vi "Digilens DLP Gen2 UI .vi"(11 "TopLevel In":refnum<class "TopLevel.lvclass">) -> (3 "TopLevel Out":refnum<class "TopLevel.lvclass">)   [LabVIEW 2022 SP3, in "TopLevel.lvclass"] (continued)
            n1054 = Unbundle By Name(w3179) -> ("Materials"=w3165:string[], "Color Panes"=w3163:string[], "DLP2Config.ColorPaneMapping.Head 1.Material"=w3178:string, "DLP2Config.ColorPaneMapping.Head 1.ColorPane"=w3172:string, "DLP2Config.ColorPaneMapping.Head 2.Material"=w3177:string, "DLP2Config.ColorPaneMapping.Head 2.ColorPane"=w3171:string, "DLP2Config.ColorPaneMapping.Head 3.Material"=w3176:string, "DLP2Config.ColorPaneMapping.Head 3.ColorPane"=w3170:string, "DLP2Config.ColorPaneMapping.Head 4.Material"=w3175:string, "DLP2Config.ColorPaneMapping.Head 4.ColorPane"=w3169:string, "DLP2Config.ColorPaneMapping.Head 5.Material"=w3174:string, "DLP2Config.ColorPaneMapping.Head 5.ColorPane"=w3168:string, "DLP2Config.ColorPaneMapping.Head 6.Material"=w3173:string, "DLP2Config.ColorPaneMapping.Head 6.ColorPane"=w3167:string)
            n1055 = Build Array(w3172, w3171, w3170, w3169, w3168, w3167) -> (w3164:string[])
            n1056 = Build Array(w3178, w3177, w3176, w3175, w3174, w3173) -> (w3166:string[])
            n1057 = for {
              tunnel: w3166 -> [w3189] mode=indexing
              tunnel: w3165 -> [w3188]
              tunnel: [w3186] -> w3161 mode=indexing
              n1058 = Search 1D Array(1D array=w3188, element=w3189) -> (index of element=w3187:i32)  [unwired: 1 in]
              n1059 = Greater Than 0?(x=w3187) -> (x > 0?=w3186:bool)
            }
            n1060 = for {
              tunnel: w3164 -> [w3185] mode=indexing
              tunnel: w3163 -> [w3184]
              tunnel: [w3182] -> w3162 mode=indexing
              n1061 = Search 1D Array(1D array=w3184, element=w3185) -> (index of element=w3183:i32)  [unwired: 1 in]
              n1062 = Greater Than 0?(x=w3183) -> (x > 0?=w3182:bool)
            }
            n1063 = And Array Elements(Boolean array=w3161) -> (logical AND=w3159:bool)
            n1064 = And Array Elements(Boolean array=w3162) -> (logical AND=w3160:bool)
            n1065 = case shown="True" w3160 {
              frame False {
              }
              frame True {
                n1066 = One Button Dialog(message="Atleast 1 material  mismatch\nbetween DB and Config") -> ()  [unwired: 1 in, 1 out]
              }
            }
            n1067 = case shown="True" w3159 {
              frame False {
              }
              frame True {
                n1068 = One Button Dialog(message="Atleast 1 ColorPlane  mismatch\nbetween DB and Config") -> ()  [unwired: 1 in, 1 out]
              }
            }
          }
          frame Enabled {
          }
        }
        n1069 = call <vilib>:"Add State(s) to Queue__JKI_lib_State_Machine.vi"("State(s) in (\"\")"=w3158) -> ("States Out"=w3157:string)  [unwired: 14 in]
      }
      frame "Data: GetMaterialsAndColorPlanes" {
        w3195 = T18[] [enum."1", enum."2", enum."3", enum."4", enum."5", enum."6"] items=["-1", "1", "2", "3", "4", "5", "6"]
        n1070 = Unbundle By Name(w3202) -> ("DLP2Config.ColorPlanes"=w3196:string[], "DLP2Config.Materials"=w3197:string[], "Database"=w3201:refnum<class "Database.lvclass">, "TopLevel out"=w3194:refnum<class "TopLevel.lvclass">)
        n1071 = property class="TopLevel.lvclass" props=["Methods:Accessors:ConfigDict", "Methods:Accessors:PrinterInitializationXML"](reference=w3194) -> ("Methods:Accessors:PrinterInitializationXML"=w3193:T61)  [unwired: 1 in, 3 out]
        n1072 = Unbundle By Name(w3193) -> ("InkSet.Ink"=w3192:T65[])  [unwired: 1 out]
        n1073 = disable-structure shown="Enabled" {
          disable-tunnel: w3201 -> [w3219 _ _]
          disable-tunnel: [w3216 w3220 w3236] -> w3200
          disable-tunnel: w3199 -> [w3215 w3220 w3230]
          disable-tunnel: [w3208 w3221 w3235] -> w3190
          disable-tunnel: [w3207 w3222 _] -> _
          disable-tunnel: w3197 -> [_ w3222 _]
          disable-tunnel: w3196 -> [_ w3221 _]
          disable-tunnel: w3194 -> [_ _ w3233]
          disable-tunnel: w3195 -> [_ _ w3237]
          disable-tunnel: w3192 -> [_ _ w3234]
          disable-tunnel: [_ _ w3231] -> w3191
          frame Disabled {
            w3213 = u32 3000 ("Timeout (ms)")
            w3214 = TRUE ("Wait (F)")
            n1074 = call "API_DB.GetAllMaterials.vi"("Database in"=w3219, "Wait (F)"=w3214, "error in (no error)"=w3215, "Timeout (ms)"=w3213) -> ("Database out"=w3218:refnum<class "Database.lvclass">, "Materials"=w3212:string[], "error out"=w3217:errorcluster)  [unwired: 9 in]
            n1075 = call "API_DB.GetAllColors.vi"("Database in"=w3218, "Wait (F)"=w3214, "error in (no error)"=w3217, "Timeout (ms)"=w3213) -> ("ColorPlanes"=w3209:string[], "error out"=w3216:errorcluster)  [unwired: 9 in, 1 out]
            n1076 = Build Array (concatenate)("none", w3212) -> (w3207:string[])
            n1077 = Build Array (concatenate)("none", w3209) -> (w3208:string[])
          }
          frame Disabled {
          }
          frame Enabled {
            n1078 = for {
              shift-right: [w3244] -> w3232
              shift-left: w3233 -> [w3245]
              shift-right: [w3242] -> w3236
              shift-left: w3230 -> [w3243]
              tunnel: [w3240] -> w3235 mode=indexing
              tunnel: w3234 -> [w3239] mode=indexing
              tunnel: [w3238] -> w3231 mode=indexing
              n1079 = Unbundle By Name(w3239) -> ("#attributes.InkType"=w3238:string)
              n1080 = call "GetMaterialPropertiesInConfigDict.vi"("error in (no error)"=w3243, "MaterialName"=w3238, "TopLevel in"=w3245) -> ("error out"=w3242:errorcluster, "Cluster"=w3241:T85, "TopLevel out"=w3244:refnum<class "TopLevel.lvclass">)  [unwired: 6 in]
              n1081 = Unbundle By Name(w3241) -> ("Ink.#attributes.ColorPlane"=w3240:string)
            }
            n1082 = property on="Head 4 Material" class="Ring (strict)"("Strings []"=w3231) -> ()  [unwired: 2 in, 2 out]
            n1083 = property on="Head 1 Material" class="Ring (strict)"("Strings []"=w3231) -> ()  [unwired: 2 in, 2 out]
            n1084 = property on="Head 5 Material" class="Ring (strict)"("Strings []"=w3231) -> ()  [unwired: 2 in, 2 out]
            n1085 = property on="Head 2 Material" class="Ring (strict)"("Strings []"=w3231) -> ()  [unwired: 2 in, 2 out]
            n1086 = property on="Head 6 Material" class="Ring (strict)"("Strings []"=w3231) -> ()  [unwired: 2 in, 2 out]
            n1087 = property on="Head 3 Material" class="Ring (strict)"("Strings []"=w3231) -> ()  [unwired: 2 in, 2 out]
            n1088 = property on="Head 4 Material 2" class="Ring (strict)"("Strings []"=w3231) -> ()  [unwired: 2 in, 2 out]
            n1089 = property on="Head 6 Material 2" class="Ring (strict)"("Strings []"=w3231) -> ()  [unwired: 2 in, 2 out]
            n1090 = property on="Head 1 Material 2" class="Ring (strict)"("Strings []"=w3231) -> ()  [unwired: 2 in, 2 out]
            n1091 = property on="Head 2 Material 2" class="Ring (strict)"("Strings []"=w3231) -> ()  [unwired: 2 in, 2 out]
            n1092 = property on="Head 3 Material 2" class="Ring (strict)"("Strings []"=w3231) -> ()  [unwired: 2 in, 2 out]
            n1093 = property on="Head 5 Material 2" class="Ring (strict)"("Strings []"=w3231) -> ()  [unwired: 2 in, 2 out]
            n1094 = for {
              shift-right: [w3254] -> _
              shift-left: w3232 -> [w3255]
              tunnel: w3237 -> [w3250] mode=indexing
              shift-right: [w3252] -> _
              shift-left: _ -> [w3253]
              tunnel: w3231 -> [w3249]
              tunnel: [w3247] -> _ mode=indexing
              tunnel: [w3246] -> w3229 mode=indexing
              n1095 = call "GetHeadPropertiesInConfigDict.vi"("error in (no error)"=w3253, "#attributes.HeadNumber"=w3250, "TopLevel in"=w3255) -> ("error out"=w3252:errorcluster, "HeadProperties"=w3251:T63, "TopLevel out"=w3254:refnum<class "TopLevel.lvclass">)  [unwired: 6 in]
              n1096 = Unbundle By Name(w3251) -> ("#attributes.Material"=w3248:string)
              n1097 = Search 1D Array(1D array=w3249, element=w3248) -> (index of element=w3246:i32)  [unwired: 1 in]
              n1098 = Greater Or Equal To 0?(x=w3246) -> (x >= 0?=w3247:bool)
            }
            n1099 = Index Array(array=w3229) -> (element #1=w3228:i32, element #2=w3227:i32, element #3=w3226:i32, element #4=w3225:i32, element #5=w3224:i32, element #6=w3223:i32)  [unwired: 6 in]
            n1100 = property on="Head 4 Material 2" class="Ring (strict)"("Value"=w3225) -> ()  [unwired: 2 in, 2 out]
            n1101 = property on="Head 6 Material 2" class="Ring (strict)"("Value"=w3223) -> ()  [unwired: 2 in, 2 out]
            n1102 = property on="Head 1 Material 2" class="Ring (strict)"("Value"=w3228) -> ()  [unwired: 2 in, 2 out]
            n1103 = property on="Head 2 Material 2" class="Ring (strict)"("Value"=w3227) -> ()  [unwired: 2 in, 2 out]
            n1104 = property on="Head 3 Material 2" class="Ring (strict)"("Value"=w3226) -> ()  [unwired: 2 in, 2 out]
            n1105 = property on="Head 5 Material 2" class="Ring (strict)"("Value"=w3224) -> ()  [unwired: 2 in, 2 out]
            n1106 = property on="Head 1 Material" class="Ring (strict)"("Value"=w3228) -> ()  [unwired: 2 in, 2 out]
            n1107 = property on="Head 2 Material" class="Ring (strict)"("Value"=w3227) -> ()  [unwired: 2 in, 2 out]
            n1108 = property on="Head 3 Material" class="Ring (strict)"("Value"=w3226) -> ()  [unwired: 2 in, 2 out]
            n1109 = property on="Head 4 Material" class="Ring (strict)"("Value"=w3225) -> ()  [unwired: 2 in, 2 out]
            n1110 = property on="Head 5 Material" class="Ring (strict)"("Value"=w3224) -> ()  [unwired: 2 in, 2 out]
            n1111 = property on="Head 6 Material" class="Ring (strict)"("Value"=w3223) -> ()  [unwired: 2 in, 2 out]
          }
        }
        n1112 = Bundle By Name(cluster=w3202, "DLP2Config.Materials"=w3191, "Color Panes"=w3190) -> (w3198:T77)
        n1113 = property on="Head 4 ColorPlane" class="Ring (strict)"("Strings []"=w3190) -> ()  [unwired: 2 in, 2 out]
        n1114 = property on="Head 1 ColorPlane" class="Ring (strict)"("Strings []"=w3190) -> ()  [unwired: 2 in, 2 out]
        n1115 = property on="Head 2 ColorPlane" class="Ring (strict)"("Strings []"=w3190) -> ()  [unwired: 2 in, 2 out]
        n1116 = property on="Head 3 ColorPlane" class="Ring (strict)"("Strings []"=w3190) -> ()  [unwired: 2 in, 2 out]
        n1117 = property on="Head 6 ColorPlane" class="Ring (strict)"("Strings []"=w3190) -> ()  [unwired: 2 in, 2 out]
        n1118 = property on="Head 5 ColorPlane" class="Ring (strict)"("Strings []"=w3190) -> ()  [unwired: 2 in, 2 out]
        n1119 = call <vilib>:"Add State(s) to Queue__JKI_lib_State_Machine.vi"("State(s) in (\"\")"=w3206) -> ("States Out"=w3205:string)  [unwired: 14 in]
      }
      frame "Data: Initialize" {
        w3256 = path[] []  # PPP_Ditherered_Images
        w3257 = FALSE  # PrePrimeTmrEnabled
        w3258 = TRUE  # PrePrimeDone
        w3260 = T75 {"UserLevel"=enum."Operator", "Login Time"=timestamp(0 s since 1904-01-01)}  # Login
        w3261 = T74 {"CellPrintRecipe"={"#attributes"={"Type"="", "RecipeName"="", "Product"=""}, "CellPrint"=[], "InkCompensationSet"={"InkCompensation"=[]}}}  # CalibrationPrints
        w3262 = T73 {"CellPrintRecipe"={"#attributes"={"Type"="", "RecipeName"="", "Product"=""}, "CellPrint"=[], "InkCompensationSet"={"InkCompensation"=[]}}}  # CurrentDLPRecipe
        w3263 = T71 {"PH1_Enable"=FALSE, "PH2_Enable"=FALSE, "PH3_Enable"=FALSE, "PH4_Enable"=FALSE, "PH5_Enable"=FALSE, "PH6_Enable"=FALSE}  # HeadStatusPollData
        w3269 = T49 {"Path_to_Tiff"=path "", "OutputFolder"=path "", "DPI_x"=0, "DPI_y"=0, "Python_Version"=enum."3.9 32"}  # SeparateLayers
        w3270 = T68 {"Path"=path "", "Type"="", "Product"=""}  # PrintDesign
        w3271 = cluster{"RecipeXMLPath":path} {"RecipeXMLPath"=path ""}  # Print
        w3275 = T71 {"PH1_Enable"=FALSE, "PH2_Enable"=FALSE, "PH3_Enable"=FALSE, "PH4_Enable"=FALSE, "PH5_Enable"=FALSE, "PH6_Enable"=FALSE}  # HeadStatus
        w3276 = variant  # SettingsUpdate
        w3277 = T70[] []  # GISHeadStatus
        w3278 = T86 {"Head 1"={"Actual"=0.0, "Target"=0.0}, "Head 2"={"Actual"=0.0, "Target"=0.0}, "Head 3"={"Actual"=0.0, "Target"=0.0}, "Head 4"={"Actual"=0.0, "Target"=0.0}, "Head 5"={"Actual"=0.0, "Target"=0.0}, "Head 6"={"Actual"=0.0, "Target"=0.0}}  # Head Temp
        w3279 = cluster{"HeaterEnblHead":T18, "Enable":bool} {"HeaterEnblHead"=enum."1", "Enable"=FALSE}  # Heater Enable
        w3282 = T69 {"ImageBufferMain"=[], "ChannelTargetMaterials"=[], "MaterialNames"=[]}  # TIFFImageData
        w3283 = T6 refnum  # Planes Image
        w3284 = T6 refnum  # RGB Image
        w3285 = refnum<class "DAQ.lvclass"> refnum  # DAQ
        w3294 = FALSE  # ConfigSaveRequired
        w3295 = string[] []  # Color Panes
        w3296 = string[] []  # Materials
        w3300 = refnum<class "DLP2.lvclass"> refnum  # DLP2
        w3299 = refnum<class "Database.lvclass"> refnum  # Database
        w3303 = API_Command_Enum."Execute Printer Commands"  # API Command
        w3304 = T67 {"GIS File Path"=path "", "Duration (s)"=0.1, "No. of Repeats"=1}  # Pre Purge Parameters
        w3305 = ICP1-D0_Channel_Names."None"  # Purge\PrePurge Channel Name
        w3312 = refnum<class "Motor Controller.lvclass"> refnum  # Motor Controller
        w3315 = refnum<class "GIS Printer.lvclass"> refnum  # GIS Printer
        w3317 = refnum<class "IO.lvclass"> refnum  # IO
        w3322 = T87 {"Current VI Reference"=refnum, "Close Panel on Exit?"=FALSE}  # Core
        n1120 = property class="TopLevel.lvclass"(reference=w3321) -> (reference out=w3309:refnum<class "TopLevel.lvclass">, "Methods:Accessors:IO"=w3319:refnum<class "IO.lvclass">, "Methods:Accessors:GIS Printer"=w3320:refnum<class "GIS Printer.lvclass">, "Methods:Accessors:Motor Controller"=w3314:refnum<class "Motor Controller.lvclass">, "Methods:Accessors:Digilens Config"=w3293:T51, "Methods:Accessors:PrinterInitializationXML"=w3274:T61, "Methods:Accessors:Database"=w3302:refnum<class "Database.lvclass">, "Methods:Accessors:DLP2"=w3301:refnum<class "DLP2.lvclass">, "Methods:Accessors:DLP2Config"=w3289:T35, "Methods:Accessors:DAQ"=w3287:refnum<class "DAQ.lvclass">, "Methods:Accessors:ConfigDict"=w3273:T16)  [unwired: 1 in, 1 out]
        n1121 = call-dynamic "GetEvents_TopLevel.vi"("error in (no error)"=w3307, "TopLevel in"=w3309) -> ("error out"=w3266:errorcluster, "UserEvents"=w3308:T88, "TopLevel out"=w3268:refnum<class "TopLevel.lvclass">)  [unwired: 7 in]
        n1122 = call-dynamic "Read PersistentXML.vi"("error in (no error)"=w3266, "TopLevel in"=w3268) -> ("error out"=w3265:errorcluster, "PersistentData"=w3264:T72, "TopLevel out"=w3267:refnum<class "TopLevel.lvclass">)  [unwired: 7 in]
        n1123 = Coerce To Type(0:w3289, 1:T35 {"Paths"={"DigiBit WG Design Folder"=path "", "Compensated GS Image Folder"=path "", "Nozzle GS Files Head 1"=path "", "Nozzle GS Files Head 2"=path "", "Nozzle GS Files Head 3"=path "", "Nozzle GS Files Head 4"=path "", "Nozzle GS Files Head 5"=path "", "Nozzle GS Files Head 6"=path ""}, "ColorPaneMapping"={"Head 1"={"Material"="", "ColorPane"=""}, "Head 2"={"Material"="", "ColorPane"=""}, "Head 3"={"Material"="", "ColorPane"=""}, "Head 4"={"Material"="", "ColorPane"=""}, "Head 5"={"Material"="", "ColorPane"=""}, "Head 6"={"Material"="", "ColorPane"=""}}, "Materials"=[], "ColorPlanes"=[], "SpitVoltages_Half"={"1"=0.0, "2"=0.0, "3"=0.0, "4"=0.0, "5"=0.0, "6"=0.0}, "SpitVoltages_Full"={"1"=0.0, "2"=0.0, "3"=0.0, "4"=0.0, "5"=0.0, "6"=0.0}, "SystemMode"=[], "PrimeModeConfig"=[], "Running Average Duration_s"=5.0} ("DLP2ConfigLoaded")) -> (2:w3288:T35)
        n1124 = Coerce To Type(0:w3289, 1:T35 {"Paths"={"DigiBit WG Design Folder"=path "", "Compensated GS Image Folder"=path "", "Nozzle GS Files Head 1"=path "", "Nozzle GS Files Head 2"=path "", "Nozzle GS Files Head 3"=path "", "Nozzle GS Files Head 4"=path "", "Nozzle GS Files Head 5"=path "", "Nozzle GS Files Head 6"=path ""}, "ColorPaneMapping"={"Head 1"={"Material"="", "ColorPane"=""}, "Head 2"={"Material"="", "ColorPane"=""}, "Head 3"={"Material"="", "ColorPane"=""}, "Head 4"={"Material"="", "ColorPane"=""}, "Head 5"={"Material"="", "ColorPane"=""}, "Head 6"={"Material"="", "ColorPane"=""}}, "Materials"=[], "ColorPlanes"=[], "SpitVoltages_Half"={"1"=0.0, "2"=0.0, "3"=0.0, "4"=0.0, "5"=0.0, "6"=0.0}, "SpitVoltages_Full"={"1"=0.0, "2"=0.0, "3"=0.0, "4"=0.0, "5"=0.0, "6"=0.0}, "SystemMode"=[], "PrimeModeConfig"=[], "Running Average Duration_s"=5.0} ("DLP2Config")) -> (2:w3291:T35)
        n1125 = Unbundle By Name(w3308) -> ("Exit Event"=w3306:refnum<user-event>)
        n1126 = Coerce To Type(0:w3319, 1:w3317) -> (2:w3318:refnum<class "IO.lvclass">)
        n1127 = Coerce To Type(0:w3287, 1:w3285) -> (2:w3286:refnum<class "DAQ.lvclass">)
        n1128 = Coerce To Type(0:w3320, 1:w3315) -> (2:w3316:refnum<class "GIS Printer.lvclass">)
        n1129 = Coerce To Type(0:w3302, 1:w3299) -> (2:w3298:refnum<class "Database.lvclass">)
        n1130 = Coerce To Type(0:w3301, 1:w3300) -> (2:w3297:refnum<class "DLP2.lvclass">)
        n1131 = call "GetPrimeConfigKeys.vi"() -> ("Prime Names"=w3272:T89)  [unwired: 11 in]
        n1132 = Coerce To Type(0:w3314, 1:w3312) -> (2:w3313:refnum<class "Motor Controller.lvclass">)
        n1133 = call <vilib>:"Add State(s) to Queue__JKI_lib_State_Machine.vi"("State(s) in (\"\")"=w3325) -> ("States Out"=w3324:string)  [unwired: 14 in]
        n1134 = Bundle("Core"=w3322, "IO"=w3318, "GIS Printer"=w3316, "Motor Controller"=w3313, "Methods:Accessors:Digilens Config"=w3293, "Methods:Accessors:PrinterInitializationXML"=w3274, "Status"=T40 {"Motor Controller Config Data"={"Motor IP Addresss"="", "Current Position"=0, "Pulse_Per_mm"=0, "PrePrint"=[], "Load Position_mm"=0, "Laminate Position_mm"=0}, "Motor Controller Data"={"Enabled?"=FALSE}, "Stage Move"={"Current Step"="", "Move Data"=[]}, "Stage Busy?"=FALSE}, "Exit Event"=w3306, "Purge\\PrePurge Channel Name"=w3305, "Pre Purge Parameters"=w3304, "API Command"=w3303, "TopLevel out"=w3267, "Database"=w3298, "DLP2"=w3297, "DLP2Config"=w3291, "Materials"=w3296, "Color Panes"=w3295, "ConfigSaveRequired"=w3294, "DLP2ConfigLoaded"=w3288, "PrintDesign"=w3270, "DAQ"=w3286, "RGB Image"=w3284, "Planes Image"=w3283, "TIFFImageData"=w3282, "Image Resolution"=T34 {"X Resolution"=0, "Y Resolution"=0}, "Pre Purge API Data"=T27 {"Interval (s)"=0.1, "PurgeDuration (s)"=0.1, "Repeats"=0, "PrimingMode"=enum."Pre-Purge", "Head"=enum."1", "Frequency (Hz)"=0, "PrintWeight"=0.1}, "Prime Names"=w3272, "Heater Enable"=w3279, "Head Temp"=w3278, "GISHeadStatus"=w3277, "SettingsUpdate"=w3276, "HeadStatus"=w3275, "Methods:Accessors:ConfigDict"=w3273, "Print"=w3271, "SeparateLayers"=w3269, "PersistentData"=w3264, "HeadStatusPollData"=w3263, "CurrentDLPRecipe"=w3262, "CalibrationPrints"=w3261, "Login"=w3260, "PrintWeights"=T33 {"Weights 1"=0.3, "Weights 2"=0.3, "Weights 3"=0.3, "Weights 4"=0.3, "Weights 5"=0.3, "Weights 6"=0.3}, "PrePrimeDone"=w3258, "PrePrimeTmrEnabled"=w3257, "PPP_Ditherered_Images"=w3256) -> (w3323:T77)  [unwired: 1 in]
      }
      frame "Data: Create Images" {
        w3328 = T90 0 items=["Grayscale (U8)", "Grayscale (I16)", "Grayscale (SGL)", "Complex (CSG)", "RGB (U32)", "HSL (U32)", "RGB (U64)", "Grayscale (U16)"] ("Image Type")
        w3334 = T90 4 items=["Grayscale (U8)", "Grayscale (I16)", "Grayscale (SGL)", "Complex (CSG)", "RGB (U32)", "HSL (U32)", "RGB (U64)", "Grayscale (U16)"] ("Image Type")
        n1135 = call "IMAQ Create"("Image Name"="RGB_TIFF_Image", "Image Type"=w3334, "error in (no error)"=w3333) -> ("New Image"=w3331:T6, "error out"=w3330:errorcluster)  [unwired: 2 in]
        n1136 = call "IMAQ Create"("Image Name"="TIFF_Planes_Image" ("String"), "Image Type"=w3328, "error in (no error)"=w3330) -> ("New Image"=w3327:T6, "error out"=w3329:errorcluster)  [unwired: 2 in]
        n1137 = Bundle By Name(cluster=w3338, "RGB Image"=w3331, "Planes Image"=w3327) -> (w3332:T77)
      }
      frame "Data: Cleanup" {
        # "Cleanup any data and references, here.\n(this is called automatically, by the Macro: Exit)"
        n1138 = Unbundle By Name(w3346) -> ("Core.Current VI Reference"=w3349:refnum<vi>, "Planes Image"=w3343:T6, "RGB Image"=w3342:T6)
        n1139 = call "IMAQ Dispose"("Image"=w3342) -> ("error out"=w3340:errorcluster)  [unwired: 5 in]
        n1140 = call "IMAQ Dispose"("Image"=w3343) -> ("error out"=w3341:errorcluster)  [unwired: 5 in]
        n1141 = flat-sequence {
          tunnel: w3341 -> [_]
          tunnel: w3340 -> [_]
          frame #0 {
          }
        }
        n1142 = Close Reference(reference=w3349, error in (no error)=w3348) -> (error out=w3347:errorcluster)
        n1143 = call <vilib>:"Add State(s) to Queue__JKI_lib_State_Machine.vi"("State(s) in (\"\")"=w3351) -> ("States Out"=w3350:string)  [unwired: 14 in]
      }
      frame "---------- UI ----------" {
        n1144 = call <vilib>:"Add State(s) to Queue__JKI_lib_State_Machine.vi"("State(s) in (\"\")"=w3357) -> ("States Out"=w3356:string)  [unwired: 14 in]
      }
      frame "UI: Update Status" {
        n1145 = control-ref of="PrintStatus"() -> (w3359:refnum<vi>)
        n1146 = property class="Str"(reference=w3359, "Value"=w3358) -> ()  [unwired: 1 in, 2 out]
        n1147 = call <vilib>:"Add State(s) to Queue__JKI_lib_State_Machine.vi"("State(s) in (\"\")"=w3365) -> ("States Out"=w3364:string)  [unwired: 14 in]
      }
      frame "UI: PrimeHeadTimerInit" {
        n1148 = property on="EnableHeadPrimeTimer" class="Bool (strict)"("Value"=TRUE ("Value (Signaling)")) -> ()  [unwired: 2 in, 2 out]
        n1149 = call <vilib>:"Add State(s) to Queue__JKI_lib_State_Machine.vi"("State(s) in Front (\"\")"="Action: PrePrimeTimer>>Init\nUI: EnableControls>>PrimeHeads>>True\nUI: EnableControls>>Print PPP Image>>False" ("State(s) in Front (\"\")"), "State(s) in (\"\")"=w3373) -> ("States Out"=w3372:string)  [unwired: 13 in]
      }
      frame "UI: Process Head Enabled Mode" {
        n1150 = Unbundle By Name(w3383) -> ("TopLevel out"=w3376:refnum<class "TopLevel.lvclass">)
        n1151 = call "FindEnable_DisableStatus.vi"("TopLevel in"=w3376) -> ("error out"=w3381:errorcluster, "Array"=w3382:T91)  [unwired: 8 in, 1 out]
        n1152 = Index Array(array=w3382) -> (element #1=w3377:T45, element #2=w3378:T45, element #3=w3379:T45, element #4=w3380:T45, element #5=w3375:T45, element #6=w3374:T45)  [unwired: 6 in]
        n1153 = property on="PrinterControls 5" class="TabCtl (strict)"("DisabledEnum"=w3375) -> ()  [unwired: 2 in, 2 out]
        n1154 = property on="PrinterControls 6" class="TabCtl (strict)"("DisabledEnum"=w3374) -> ()  [unwired: 2 in, 2 out]
        n1155 = property on="PrinterControls 4" class="TabCtl (strict)"("DisabledEnum"=w3380) -> ()  [unwired: 2 in, 2 out]
        n1156 = property on="PrinterControls 3" class="TabCtl (strict)"("DisabledEnum"=w3379) -> ()  [unwired: 2 in, 2 out]
        n1157 = property on="PrinterControls" class="TabCtl (strict)"(error in=w3381, "DisabledEnum"=w3377) -> ()  [unwired: 1 in, 2 out]
        n1158 = property on="PrinterControls 2" class="TabCtl (strict)"("DisabledEnum"=w3378) -> ()  [unwired: 2 in, 2 out]
        n1159 = property on="MinCtrl 1" class="TabCtl (strict)"("DisabledEnum"=w3377) -> ()  [unwired: 2 in, 2 out]
        n1160 = property on="MinCtrl 2" class="TabCtl (strict)"("DisabledEnum"=w3378) -> ()  [unwired: 2 in, 2 out]
        n1161 = property on="MinCtrl 3" class="TabCtl (strict)"("DisabledEnum"=w3379) -> ()  [unwired: 2 in, 2 out]
        n1162 = property on="MinCtrl 4" class="TabCtl (strict)"("DisabledEnum"=w3380) -> ()  [unwired: 2 in, 2 out]
        n1163 = property on="MinCtrl 5" class="TabCtl (strict)"("DisabledEnum"=w3375) -> ()  [unwired: 2 in, 2 out]
        n1164 = property on="MinCtrl 6" class="TabCtl (strict)"("DisabledEnum"=w3374) -> ()  [unwired: 2 in, 2 out]
        n1165 = property on="Dig H 5" class="TabCtl (strict)"("DisabledEnum"=w3375) -> ()  [unwired: 2 in, 2 out]
        n1166 = property on="Dig H 6" class="TabCtl (strict)"("DisabledEnum"=w3374) -> ()  [unwired: 2 in, 2 out]
        n1167 = property on="INK H 5" class="TabCtl (strict)"("DisabledEnum"=w3375) -> ()  [unwired: 2 in, 2 out]
        n1168 = property on="INK H 6" class="TabCtl (strict)"("DisabledEnum"=w3374) -> ()  [unwired: 2 in, 2 out]
        n1169 = call <vilib>:"Add State(s) to Queue__JKI_lib_State_Machine.vi"("State(s) in (\"\")"=w3388) -> ("States Out"=w3387:string)  [unwired: 14 in]
      }
      frame "UI: Initialize" {
        n1170 = Unbundle By Name(w3441) -> ("Core.Current VI Reference"=w3444:refnum<vi>, "DLP2ConfigLoaded.SystemMode"=w3438:string[])
        n1171 = Unbundle By Name(w3441) -> ("Methods:Accessors:PrinterInitializationXML.PrinterInitialization.VacPumpSet.#attributes.VacPumpSpeed"=w3429:dbl, "Methods:Accessors:PrinterInitializationXML.PrinterInitialization.VacPumpSet.#attributes.VacPumpEnable"=w3430:bool, "Methods:Accessors:Digilens Config.PrinterConfiguration.PrintScriptsFolder"=w3440:path, "Methods:Accessors:Digilens Config.PrinterConfiguration.StageScriptsFolder"=w3439:path)
        n1172 = call <userlib>:"Fit VI window to Largest Dec__ogtk.vi"("error in (no error)"=w3417, "VI Ref (calling VI)"=w3444) -> ("error out"=w3435:errorcluster)  [unwired: 4 in, 1 out]
        n1173 = property on="TCP Commands & Responses" class="MCListbox (strict)"("ItemNames"=string[][] [] ("Item Names")) -> ()  [unwired: 2 in, 2 out]
        n1174 = property on="System Mode" class="Ring (strict)"("Strings []"=w3438) -> ()  [unwired: 2 in, 2 out]
        n1175 = case shown="True" w3430 {
          tunnel: w3429 -> [_ w3496]
          tunnel: w3428 -> [w3495 w3499]
          tunnel: [w3495 w3498] -> w3427
          frame False {
          }
          frame True {
            n1176 = local write "Meniscus Vac Pump Speed"(w3496) -> ()
            n1177 = call <vilib>:"Add State(s) to Queue__JKI_lib_State_Machine.vi"("State(s) in Front (\"\")"="Set Vacuum Pump Speed" ("State(s) in Front (\"\")"), "State(s) in (\"\")"=w3499) -> ("States Out"=w3498:string)  [unwired: 13 in]
          }
        }
        n1178 = property on="Command File Path" class="Path"("StartPath"=w3440) -> ()  [unwired: 2 in, 2 out]
        n1179 = property on="Stage Recipe XML File Path" class="Path"("StartPath"=w3439) -> ()  [unwired: 2 in, 2 out]
        n1180 = local write "Login"(FALSE ("Login")) -> ()
        n1181 = local write "Stage Recipe XML File Path"(path "" ("Recipe XML File Path")) -> ()
        n1182 = control-ref of="SettingsTabs"() -> (w3437:refnum<vi>)
        n1183 = call "Tab Control Ref.vi"("Page Label"="Digital IO" ("Page Name"), "error in"=w3435, "TabControl Reference"=w3437) -> ("error out"=w3422:errorcluster, "Array Out"=w3434:string[], "Array"=w3433:refnum<vi>[])  [unwired: 6 in]
        n1184 = for {
          tunnel: w3434 -> [w3504] mode=indexing
          shift-right: [w3503] -> w3418
          shift-left: w3431 -> [w3505]
          tunnel: w3433 -> [w3502] mode=indexing
          shift-right: [w3500] -> w3420
          shift-left: w3422 -> [w3501]
          n1185 = call <vilib>:"Set Dynamic CVT Data.vi"("error in (no error)"=w3501, "value"=w3502, "DataName"=w3504, "dCVT DVR"=w3505) -> ("error out"=w3500:errorcluster, "dCVT DVR out"=w3503:T16)  [unwired: 5 in, 1 out]
        }
        n1186 = control-ref of="MinCtrl 2"() -> (w3401:refnum<vi>)
        n1187 = control-ref of="MinCtrl 3"() -> (w3402:refnum<vi>)
        n1188 = control-ref of="MinCtrl 4"() -> (w3403:refnum<vi>)
        n1189 = control-ref of="MinCtrl 1"() -> (w3400:refnum<vi>)
        n1190 = control-ref of="MinCtrl 5"() -> (w3404:refnum<vi>)
        n1191 = control-ref of="MinCtrl 7"() -> (w3406:refnum<vi>)
        n1192 = control-ref of="MinCtrl 6"() -> (w3405:refnum<vi>)
        n1193 = disable-structure shown="Disabled" {
          frame Disabled {
            n1194 = disable-structure shown="Default" {
              disable-tunnel: [TRUE FALSE] -> w3447
              frame condition #0 (active) {
              }
              frame condition #1 {
              }
            }
            n1195 = property on="Tab Control" class="TabCtl (strict)"("PageSelVis"=w3447) -> ()  [unwired: 2 in, 2 out]
            n1196 = property on="SettingsTabs" class="TabCtl (strict)"("PageSelVis"=w3447) -> ()  [unwired: 2 in, 2 out]
          }
          frame Enabled {
          }
        }
        n1197 = control-ref of="SettingsTabs"() -> (w3425:refnum<vi>)
        n1198 = call "Tab Control Ref.vi"("Page Label"="Analog IO" ("Page Name"), "error in"=w3420, "TabControl Reference"=w3425) -> ("error out"=w3421:errorcluster, "Array Out"=w3423:string[], "Array"=w3424:refnum<vi>[])  [unwired: 6 in]
        n1199 = Build Array(w3400, w3401, w3402, w3403, w3404, w3405, w3406) -> (w3407:refnum<vi>[])
        n1200 = for {
          tunnel: w3423 -> [w3493] mode=indexing
          shift-right: [w3492] -> w3399
          shift-left: w3418 -> [w3494]
          tunnel: w3424 -> [w3491] mode=indexing
          shift-right: [w3489] -> w3419
          shift-left: w3421 -> [w3490]
          n1201 = call <vilib>:"Set Dynamic CVT Data.vi"("error in (no error)"=w3490, "value"=w3491, "DataName"=w3493, "dCVT DVR"=w3494) -> ("error out"=w3489:errorcluster, "dCVT DVR out"=w3492:T16)  [unwired: 5 in, 1 out]
        }
        n1202 = for {
          shift-right: [w3465] -> w3391
          shift-left: w3399 -> [w3464]
          tunnel: w3407 -> [w3463] mode=indexing
          n1203 = call "Tab Control Ref.vi"("Page Label"="Generic" ("Page Name"), "TabControl Reference"=w3463) -> ("error out"=w3467:errorcluster, "Array Out"=w3469:string[], "Array"=w3468:refnum<vi>[])  [unwired: 7 in]
          n1204 = for {
            tunnel: w3469 -> [w3474] mode=indexing
            shift-right: [w3473] -> w3465
            shift-left: w3464 -> [w3475]
            tunnel: w3468 -> [w3472] mode=indexing
            shift-right: [w3470] -> _
            shift-left: w3467 -> [w3471]
            n1205 = call <vilib>:"Set Dynamic CVT Data.vi"("error in (no error)"=w3471, "value"=w3472, "DataName"=w3474, "dCVT DVR"=w3475) -> ("error out"=w3470:errorcluster, "dCVT DVR out"=w3473:T16)  [unwired: 5 in, 1 out]
          }
        }
        n1206 = control-ref of="INK H 5"() -> (w3393:refnum<vi>)
        n1207 = control-ref of="INK H 4"() -> (w3394:refnum<vi>)
        n1208 = control-ref of="INK H 6"() -> (w3392:refnum<vi>)
        n1209 = control-ref of="INK H 3"() -> (w3395:refnum<vi>)
        n1210 = control-ref of="INK H 1"() -> (w3397:refnum<vi>)
        n1211 = control-ref of="INK H 2"() -> (w3396:refnum<vi>)
        n1212 = control-ref of="Dig H 4"() -> (w3412:refnum<vi>)
        n1213 = control-ref of="Dig H 5"() -> (w3413:refnum<vi>)
        n1214 = control-ref of="Dig H 2"() -> (w3410:refnum<vi>)
        n1215 = control-ref of="Dig H 6"() -> (w3414:refnum<vi>)
        n1216 = control-ref of="Dig H 3"() -> (w3411:refnum<vi>)
        n1217 = control-ref of="Dig H 1"() -> (w3409:refnum<vi>)
        n1218 = Build Array(w3397, w3396, w3395, w3394, w3393, w3392) -> (w3398:refnum<vi>[])
        n1219 = for {
          shift-right: [w3452] -> w3390
          shift-left: w3391 -> [w3451]
          tunnel: w3398 -> [w3450] mode=indexing
          n1220 = call "Tab Control Ref.vi"("Page Label"="Generic" ("Page Name"), "TabControl Reference"=w3450) -> ("error out"=w3454:errorcluster, "Array Out"=w3456:string[], "Array"=w3455:refnum<vi>[])  [unwired: 7 in]
          n1221 = for {
            tunnel: w3456 -> [w3461] mode=indexing
            shift-right: [w3460] -> w3452
            shift-left: w3451 -> [w3462]
            tunnel: w3455 -> [w3459] mode=indexing
            shift-right: [w3457] -> _
            shift-left: w3454 -> [w3458]
            n1222 = call <vilib>:"Set Dynamic CVT Data.vi"("error in (no error)"=w3458, "value"=w3459, "DataName"=w3461, "dCVT DVR"=w3462) -> ("error out"=w3457:errorcluster, "dCVT DVR out"=w3460:T16)  [unwired: 5 in, 1 out]
          }
        }
        n1223 = Build Array(w3409, w3410, w3411, w3412, w3413, w3414) -> (w3415:refnum<vi>[])
        n1224 = for {
          shift-right: [w3478] -> w3408
          shift-left: w3390 -> [w3477]
          tunnel: w3415 -> [w3476] mode=indexing
          n1225 = call "Tab Control Ref.vi"("Page Label"="Generic" ("Page Name"), "TabControl Reference"=w3476) -> ("error out"=w3480:errorcluster, "Array Out"=w3482:string[], "Array"=w3481:refnum<vi>[])  [unwired: 7 in]
          n1226 = for {
            tunnel: w3482 -> [w3487] mode=indexing
            shift-right: [w3486] -> w3478
            shift-left: w3477 -> [w3488]
            tunnel: w3481 -> [w3485] mode=indexing
            shift-right: [w3483] -> _
            shift-left: w3480 -> [w3484]
            n1227 = call <vilib>:"Set Dynamic CVT Data.vi"("error in (no error)"=w3484, "value"=w3485, "DataName"=w3487, "dCVT DVR"=w3488) -> ("error out"=w3483:errorcluster, "dCVT DVR out"=w3486:T16)  [unwired: 5 in, 1 out]
          }
        }
        n1228 = Bundle By Name(cluster=w3441, "SettingsUpdate"=w3408) -> (w3432:T77)
        n1229 = call <vilib>:"Get ALL Dynamic CVT Data.vi"("error in (no error)"=w3419, "dCVT DVR"=w3408) -> ("NameArray"=→"NameArray":string[])  [unwired: 6 in, 3 out]
      }
      frame "UI: EnableControls" {
        n1230 = call <vilib>:"Parse State Queue__JKI_lib_State_Machine.vi"("State Queue"=w3513) -> ("Current State"=w3512:string, "Arguments"=w3511:string)  [unwired: 12 in, 1 out]
        n1231 = Scan From String(input string=w3511, default 1=FALSE) -> (output 1=w3509:bool)  [unwired: 3 in, 3 out]
        n1232 = Select(t=T45."Enabled" ("Disabled"), s=w3509, f=T45."Disabled and Grayed Out" ("Disabled")) -> (s? t:f=w3507:T45)
        n1233 = while {
          tunnel: w3512 -> [w3534]
          tunnel: w3507 -> [w3533]
          shift-right: [w3532] -> _
          shift-left: _ -> [w3529]
          shift-right: [w3531] -> _
          shift-left: _ -> [w3528]
          shift-right: [w3527] -> _
          shift-left: _ -> [w3526]
          shift-right: [w3525] -> _
          shift-left: _ -> [w3524]
          shift-right: [w3523] -> _
          shift-left: _ -> [w3522]
          shift-right: [w3521] -> _
          shift-left: _ -> [w3520]
          stop <- TRUE stop-if-true
          n1234 = case shown="\"All\"" w3534 {
            tunnel: w3533 -> [_ w3541 _ _ w3555 _ w3569 w3572 w3582 w3585]
            tunnel: [w3540 w3541 w3546 w3553 w3559 w3565 w3571 w3576 w3582 w3586] -> w3532
            tunnel: [w3539 w3541 w3543 w3552 w3558 w3564 w3570 w3572 w3581 w3588] -> w3531
            tunnel: w3529 -> [w3540 _ _ w3553 w3559 w3565 w3571 w3576 _ w3586]
            tunnel: w3528 -> [w3539 _ _ w3552 w3558 w3564 w3570 _ w3581 w3588]
            tunnel: [w3538 w3541 w3545 w3551 w3557 w3563 w3569 w3575 w3580 w3587] -> w3527
            tunnel: w3526 -> [w3538 _ _ w3551 w3557 w3563 _ w3575 w3580 w3587]
            tunnel: [w3537 w3542 T45."Enabled" ("Disabled") w3550 w3556 w3562 w3568 w3574 w3579 w3585] -> w3525
            tunnel: w3524 -> [w3537 w3542 _ w3550 w3556 w3562 w3568 w3574 w3579 _]
            tunnel: [w3536 w3541 w3544 w3549 w3555 w3561 w3567 w3573 w3578 w3584] -> w3523
            tunnel: w3522 -> [w3536 _ _ w3549 _ w3561 w3567 w3573 w3578 w3584]
            tunnel: [w3535 w3541 w3543 w3548 w3554 w3560 w3566 w3572 w3577 w3583] -> w3521
            tunnel: w3520 -> [w3535 _ _ w3548 w3554 w3560 w3566 _ w3577 w3583]
            frame Default {
            }
            frame "All" {
            }
            frame "Init" {
              w3543 = T45."Disabled and Grayed Out" ("Disabled")
              n1235 = property on="Load Calibration Rx" class="Bool"() -> ("DisabledEnum"=w3544:T45)  [unwired: 2 in, 2 out]
              n1236 = property on="RIP Recipe" class="Bool"() -> ("DisabledEnum"=w3545:T45)  [unwired: 2 in, 2 out]
              n1237 = property on="Load Customer Design" class="Bool"() -> ("DisabledEnum"=w3546:T45)  [unwired: 2 in, 2 out]
            }
            frame "SeparateLayers" {
            }
            frame "Load Calibration Rx" {
            }
            frame "InvokePPP" {
            }
            frame "RIP Recipe" {
            }
            frame "Print PPP Image" {
              # "Print PPP Image has the same behavior as\nHead Print Command button"
            }
            frame "Load Customer Design" {
            }
            frame "PrimeHeads" {
            }
          }
          n1238 = property on="PrimeHeads" class="Bool"("DisabledEnum"=w3525) -> ()  [unwired: 2 in, 2 out]
          n1239 = property on="RIP Recipe" class="Bool"("DisabledEnum"=w3527) -> ()  [unwired: 2 in, 2 out]
          n1240 = property on="Load Customer Design" class="Bool"("DisabledEnum"=w3532) -> ()  [unwired: 2 in, 2 out]
          n1241 = property on="Print PPP Image" class="Bool (strict)"("DisabledEnum"=w3531) -> ()  [unwired: 2 in, 2 out]
          n1242 = property on="Head Print Command" class="Bool (strict)"("DisabledEnum"=w3521) -> ()  [unwired: 2 in, 2 out]
          n1243 = property on="Load Calibration Rx" class="Bool"("DisabledEnum"=w3523) -> ()  [unwired: 2 in, 2 out]
        }
        n1244 = call <vilib>:"Add State(s) to Queue__JKI_lib_State_Machine.vi"("State(s) in (\"\")"=w3519) -> ("States Out"=w3518:string)  [unwired: 14 in]
      }
      frame "UI: Process Login Event" {
        n1245 = Unbundle By Name(w3600) -> ("Login.UserLevel"=w3597:T76)
        n1246 = Format Into String(w3597) -> (resulting string=w3599:string)  [unwired: 3 in, 1 out]
        n1247 = Concatenate Strings("Login: " ("string"), w3599) -> (→"LogINDetail":string)
        n1248 = case shown="\"Operator\"" w3597 {
          tunnel: [w3606 w3607 w3608] -> w3591
          tunnel: [w3606 w3607 w3608] -> w3590
          tunnel: [w3606 w3607 w3608] -> w3596
          tunnel: [w3606 w3607 w3608] -> w3595
          tunnel: [w3606 w3607 w3608] -> w3594
          tunnel: [w3606 w3607 w3608] -> w3593
          tunnel: [w3606 w3607 w3608] -> w3589
          frame "None", Default {
            w3606 = T45."Disabled and Grayed Out" ("Disabled")
          }
          frame "Operator" {
            w3607 = T45."Disabled and Grayed Out" ("Disabled")
          }
          frame "Engineer" {
            w3608 = T45."Enabled" ("Disabled")
          }
        }
        n1249 = property on="Head 4 Material 2" class="Ring (strict)"("DisabledEnum"=w3595) -> ()  [unwired: 2 in, 2 out]
        n1250 = property on="Head 6 Material 2" class="Ring (strict)"("DisabledEnum"=w3593) -> ()  [unwired: 2 in, 2 out]
        n1251 = property on="Head 1 Material 2" class="Ring (strict)"("DisabledEnum"=w3591) -> ()  [unwired: 2 in, 2 out]
        n1252 = property on="Head 2 Material 2" class="Ring (strict)"("DisabledEnum"=w3590) -> ()  [unwired: 2 in, 2 out]
        n1253 = property on="Head 3 Material 2" class="Ring (strict)"("DisabledEnum"=w3596) -> ()  [unwired: 2 in, 2 out]
        n1254 = property on="Head 5 Material 2" class="Ring (strict)"("DisabledEnum"=w3594) -> ()  [unwired: 2 in, 2 out]
        n1255 = property on="EnableHeadPrimeTimer" class="Bool (strict)"("DisabledEnum"=w3589) -> ()  [unwired: 2 in, 2 out]
        n1256 = property on="SaveINIXML" class="Bool"("DisabledEnum"=w3589) -> ()  [unwired: 2 in, 2 out]
        n1257 = property on="Print Speed" class="DigNum (strict)"("DisabledEnum"=w3590) -> ()  [unwired: 2 in, 2 out]
        n1258 = property on="Jog Speed" class="DigNum (strict)"("DisabledEnum"=w3591) -> ()  [unwired: 2 in, 2 out]
        n1259 = property on="Weights 3" class="DigNum (strict)"("DisabledEnum"=w3589) -> ()  [unwired: 2 in, 2 out]
        n1260 = property on="Weights 4" class="DigNum (strict)"("DisabledEnum"=w3589) -> ()  [unwired: 2 in, 2 out]
        n1261 = property on="Weights 1" class="DigNum (strict)"("DisabledEnum"=w3589) -> ()  [unwired: 2 in, 2 out]
        n1262 = property on="Weights 2" class="DigNum (strict)"("DisabledEnum"=w3589) -> ()  [unwired: 2 in, 2 out]
        n1263 = property on="Weights 5" class="DigNum (strict)"("DisabledEnum"=w3589) -> ()  [unwired: 2 in, 2 out]
        n1264 = property on="Weights 6" class="DigNum (strict)"("DisabledEnum"=w3589) -> ()  [unwired: 2 in, 2 out]
        n1265 = property on="Freq 6" class="DigNum (strict)"("DisabledEnum"=w3589) -> ()  [unwired: 2 in, 2 out]
        n1266 = property on="Freq 5" class="DigNum (strict)"("DisabledEnum"=w3589) -> ()  [unwired: 2 in, 2 out]
        n1267 = property on="Freq 3" class="DigNum (strict)"("DisabledEnum"=w3589) -> ()  [unwired: 2 in, 2 out]
        n1268 = property on="Freq 4" class="DigNum (strict)"("DisabledEnum"=w3589) -> ()  [unwired: 2 in, 2 out]
        n1269 = property on="Freq 2" class="DigNum (strict)"("DisabledEnum"=w3589) -> ()  [unwired: 2 in, 2 out]
        n1270 = property on="Freq 1" class="DigNum (strict)"("DisabledEnum"=w3589) -> ()  [unwired: 2 in, 2 out]
        n1271 = call <vilib>:"Add State(s) to Queue__JKI_lib_State_Machine.vi"("State(s) in (\"\")"=w3605) -> ("States Out"=w3604:string)  [unwired: 14 in]
      }
      frame "UI: Request Logout" {
        n1272 = Unbundle By Name(w3612) -> ("TopLevel out"=w3611:refnum<class "TopLevel.lvclass">)
        n1273 = call "SendLogOutRequestEvent.vi"("error in (no error)"=w3609, "TopLevel in"=w3611) -> ("error out"=w3610:errorcluster)  [unwired: 8 in, 1 out]
        n1274 = call <vilib>:"Add State(s) to Queue__JKI_lib_State_Machine.vi"("State(s) in (\"\")"=w3616) -> ("States Out"=w3615:string)  [unwired: 14 in]
      }
      frame "UI: Update Calibration Heads" {
        n1275 = Unbundle By Name(w3621) -> ("CalibrationPrints.CellPrintRecipe.CellPrint"=w3620:T81)
        n1276 = for {
          tunnel: w3620 -> [w3627] mode=indexing
          tunnel: [w3628] -> w3619 mode=indexing
          n1277 = Unbundle By Name(w3627) -> ("#attributes.Head"=w3628:i32)
        }
        n1278 = call-poly <userlib>:"Sort Array__ogtk.vi"("Array in"=w3619) -> ("Sorted Array out"=w3618:i32[])  [unwired: 9 in, 1 out]
        n1279 = Number To Decimal String(number=w3618) -> (decimal integer string=w3617:string[])  [unwired: 1 in]
        n1280 = property on="PrintHead Number" class="Ring (strict)"("Strings []"=w3617) -> ()  [unwired: 2 in, 2 out]
        n1281 = call <vilib>:"Add State(s) to Queue__JKI_lib_State_Machine.vi"("State(s) in (\"\")"=w3626) -> ("States Out"=w3625:string)  [unwired: 14 in]
      }
      frame "UI: Init Recipe Dropdowns" {
        n1282 = flat-sequence {
          tunnel: [w3638] -> w3630
          tunnel: w3630 -> [w3641]
          tunnel: [w3640] -> w3629
          tunnel: w3629 -> [w3647]
          frame #0 {
            n1283 = property on="RecipeType" class="Ring (strict)"("Val(Sgnl)"=u16 0 ("Value (Signaling)")) -> (error out=w3638:errorcluster)  [unwired: 2 in, 1 out]
          }
          frame #1 {
            n1284 = disable-structure shown="Disabled" {
              disable-tunnel: w3641 -> [w3645 _]
              disable-tunnel: [w3642 _] -> w3640
              frame Disabled {
                n1285 = call <userlib>:"Wait (ms)__ogtk.vi"("error in (no error)"=w3645, "milliseconds to wait"=u32 200) -> ("error out"=w3644:errorcluster)  [unwired: 8 in, 1 out]
                n1286 = property on="Product" class="Ring (strict)"(error in=w3644, "Val(Sgnl)"=u16 0 ("Value (Signaling)")) -> (error out=w3642:errorcluster)  [unwired: 1 in, 1 out]
              }
              frame Enabled {
              }
            }
          }
          frame #2 {
            n1287 = disable-structure shown="Disabled" {
              disable-tunnel: w3647 -> [w3649 _]
              frame Disabled {
                n1288 = call <userlib>:"Wait (ms)__ogtk.vi"("error in (no error)"=w3649, "milliseconds to wait"=u32 200) -> ("error out"=w3648:errorcluster)  [unwired: 8 in, 1 out]
                n1289 = property on="RecipeType" class="Ring (strict)"(error in=w3648, "Val(Sgnl)"=u16 0 ("Value (Signaling)")) -> ()  [unwired: 1 in, 2 out]
              }
              frame Enabled {
              }
            }
          }
        }
        n1290 = call <vilib>:"Add State(s) to Queue__JKI_lib_State_Machine.vi"("State(s) in Front (\"\")"="UI: EnableControls>>RIP Recipe>>True\nUI: EnableControls>>Print PPP Image>>False\nUI: EnableControls>>Load Calibration Rx>>True\nUI: EnableControls>>Head Print Command>>False" ("State(s) in Front (\"\")"), "State(s) in (\"\")"=w3637) -> ("States Out"=w3636:string)  [unwired: 13 in]
      }
      frame "UI: Verify and Apply Recipe Details" {
        n1291 = Unbundle By Name(w3658) -> ("TopLevel out"=w3655:refnum<class "TopLevel.lvclass">, "PrintDesign.Type"=w3657:string, "CurrentDLPRecipe"=w3656:T73)
        n1292 = case shown="\"PrintDesign\"" w3657 {
          tunnel: w3656 -> [_ w3674]
          tunnel: w3655 -> [_ w3668]
          tunnel: w3653 -> [w3663 w3666]
          tunnel: [w3663 w3665] -> w3654
          tunnel: [_ w3664] -> w3652
          frame "False", Default {
          }
          frame "PrintDesign" {
            n1293 = Unbundle By Name(w3674) -> ("CellPrintRecipe.CellPrint"=w3673:T92)
            n1294 = Index Array(array=w3673) -> (element=w3672:T93)  [unwired: 1 in]
            n1295 = Unbundle By Name(w3672) -> ("#attributes.PrintMode"=w3667:string)
            n1296 = property on="System Mode" class="Ring (strict)"() -> ("Strings []"=w3671:string[])  [unwired: 2 in, 2 out]
            n1297 = Search 1D Array(1D array=w3671, element=w3667) -> (index of element=w3670:i32)  [unwired: 1 in]
            n1298 = Greater Or Equal To 0?(x=w3670) -> (x >= 0?=w3669:bool)
            n1299 = case shown="True" w3669 {
              tunnel: w3668 -> [_ w3680]
              tunnel: w3667 -> [_ w3679]
              tunnel: w3666 -> [w3676 w3678]
              tunnel: [w3676 w3677] -> w3665
              frame False {
              }
              frame True {
                n1300 = call-dynamic "SetSystemMode API.vi"("error in (no error)"=w3678, "SystemMode"=w3679, "TopLevel in"=w3680) -> ("error out"=w3677:errorcluster)  [unwired: 7 in, 1 out]
              }
            }
            n1301 = case shown="No Error" w3665 {
              tunnel: ["UI: EnableControls>>Load Customer Design>>False" ("DictName") _] -> w3664
              frame No Error {
              }
              frame Error {
              }
            }
          }
        }
        n1302 = call <vilib>:"Add State(s) to Queue__JKI_lib_State_Machine.vi"("State(s) in Front (\"\")"=w3652, "State(s) in (\"\")"=w3662) -> ("States Out"=w3661:string)  [unwired: 13 in]
      }
      frame "UI: Update GIS Controls" {
        n1303 = Unbundle By Name(w3701) -> ("HeadStatus"=w3687:T71, "GISHeadStatus"=w3700:T70[])
        n1304 = Unbundle By Name(w3687) -> ("PH1_Enable"=w3686:bool, "PH2_Enable"=w3685:bool, "PH3_Enable"=w3684:bool, "PH4_Enable"=w3683:bool, "PH5_Enable"=w3682:bool, "PH6_Enable"=w3681:bool)
        n1305 = Index Array(array=w3700) -> (element #1=w3699:T70, element #2=w3698:T70, element #3=w3697:T70, element #4=w3696:T70, element #5=w3695:T70, element #6=w3694:T70)  [unwired: 6 in]
        n1306 = local write "Enable Ink Ch-1"(w3686) -> ()
        n1307 = local write "Enable Ink Ch-2"(w3685) -> ()
        n1308 = local write "Enable Ink Ch-3"(w3684) -> ()
        n1309 = local write "Enable Ink Ch-4"(w3683) -> ()
        n1310 = local write "Enable Ink Ch-5"(w3682) -> ()
        n1311 = local write "Enable Ink Ch-6"(w3681) -> ()
        n1312 = Unbundle By Name(w3698) -> ("HeaterEnabled"=w3692:bool)
        n1313 = Unbundle By Name(w3697) -> ("HeaterEnabled"=w3691:bool)
        n1314 = Unbundle By Name(w3699) -> ("HeaterEnabled"=w3693:bool)
        n1315 = Unbundle By Name(w3696) -> ("HeaterEnabled"=w3690:bool)
        n1316 = Unbundle By Name(w3695) -> ("HeaterEnabled"=w3689:bool)
        n1317 = Unbundle By Name(w3694) -> ("HeaterEnabled"=w3688:bool)
        n1318 = local write "Heater-1 Off 2"(w3693) -> ()
        n1319 = local write "Heater-2 Off 2"(w3692) -> ()
        n1320 = local write "Heater-3 Off 2"(w3691) -> ()
        n1321 = local write "Heater-5 Off 2"(w3689) -> ()
        n1322 = local write "Heater-6 Off 2"(w3688) -> ()
        n1323 = local write "Heater-4 Off 2"(w3690) -> ()
        n1324 = call <vilib>:"Add State(s) to Queue__JKI_lib_State_Machine.vi"("State(s) in (\"\")"=w3706) -> ("States Out"=w3705:string)  [unwired: 14 in]
      }
      frame "UI: Update Image Resolution" {
        n1325 = Unbundle By Name(w3711) -> ("Image Resolution.X Resolution"=w3709:i32, "Image Resolution.Y Resolution"=w3708:i32)
        n1326 = local read "ImageResolution"() -> (w3710:T4)
        n1327 = case shown="\"inches\"" w3710 {
          tunnel: w3709 -> [w3719 w3728 w3740]
          tunnel: w3708 -> [w3718 w3727 w3739]
          tunnel: [w3717 w3725 w3737] -> w3707
          frame "pixels", Default {
            n1328 = Format Into String(format string="%d X %d", w3719, w3718) -> (resulting string=w3717:string)  [unwired: 2 in, 1 out]
          }
          frame "mm" {
            n1329 = Multiply(x=w3728, y=0.0705) -> (x*y=w3722:dbl)
            n1330 = Multiply(x=w3727, y=0.0705) -> (x*y=w3721:dbl)
            n1331 = Format Into String(format string="%f X %f", w3722, w3721) -> (resulting string=w3725:string)  [unwired: 2 in, 1 out]
          }
          frame "inches" {
            n1332 = Multiply(x=w3740, y=0.0705) -> (x*y=w3734:dbl)
            n1333 = Multiply(x=w3739, y=0.0705) -> (x*y=w3733:dbl)
            n1334 = Divide(x=w3734, y=25.4) -> (x/y=w3732:dbl)
            n1335 = Divide(x=w3733, y=25.4) -> (x/y=w3730:dbl)
            n1336 = Format Into String(format string="%f X %f", w3732, w3730) -> (resulting string=w3737:string)  [unwired: 2 in, 1 out]
          }
        }
        "Resolution" <- w3707
        n1337 = call <vilib>:"Add State(s) to Queue__JKI_lib_State_Machine.vi"("State(s) in (\"\")"=w3716) -> ("States Out"=w3715:string)  [unwired: 14 in]
      }
      frame "UI: CheckConfigRequired" {
        n1338 = Unbundle By Name(w3745) -> ("ConfigSaveRequired"=w3744:bool)
        n1339 = Select(t=T45."Enabled" ("Disabled"), s=w3744, f=T45."Disabled and Grayed Out" ("Disabled")) -> (s? t:f=w3741:T45)
        n1340 = property on="Apply DLP GUI Config" class="Bool"("DisabledEnum"=w3741) -> ()  [unwired: 2 in, 2 out]
        n1341 = call <vilib>:"Add State(s) to Queue__JKI_lib_State_Machine.vi"("State(s) in (\"\")"=w3750) -> ("States Out"=w3749:string)  [unwired: 14 in]
      }
      frame "UI: Update DLP GUI from Config" {
        n1342 = disable-structure shown="Enabled" {
          disable-tunnel: w3751 -> [w3762 _]
          frame Disabled {
            n1343 = Unbundle By Name(w3762) -> ("DLP2Config.Paths.DigiBit WG Design Folder"=w3760:path, "DLP2Config.Paths.Compensated GS Image Folder"=w3761:path, "DLP2Config.ColorPaneMapping.Head 1.Material"=w3759:string, "DLP2Config.ColorPaneMapping.Head 2.Material"=w3758:string, "DLP2Config.ColorPaneMapping.Head 3.Material"=w3757:string)  [unwired: 15 out]
            n1344 = local write "PRODUCT RECIPE XML FOLDER PATH"(w3761) -> ()
            n1345 = local write "INITIALIZATION FILE PATH"(w3760) -> ()
            n1346 = property on="Head 1 Material 2" class="Ring (strict)"("RingText.Text"=w3759) -> ()  [unwired: 2 in, 2 out]
            n1347 = property on="Head 3 Material 2" class="Ring (strict)"("RingText.Text"=w3757) -> ()  [unwired: 2 in, 2 out]
            n1348 = property on="Head 2 Material 2" class="Ring (strict)"("RingText.Text"=w3758) -> ()  [unwired: 2 in, 2 out]
          }
          frame Enabled {
          }
        }
        n1349 = call <vilib>:"Add State(s) to Queue__JKI_lib_State_Machine.vi"("State(s) in (\"\")"=w3756) -> ("States Out"=w3755:string)  [unwired: 14 in]
      }
      frame "UI: UpatePrinterPage" {
        n1350 = Unbundle By Name(w3775) -> ("DLP2Config.ColorPaneMapping.Head 1.ColorPane"=→"H1ColorPlane":string, "DLP2Config.ColorPaneMapping.Head 2.ColorPane"=→"H2ColorPlane":string, "DLP2Config.ColorPaneMapping.Head 3.ColorPane"=→"H3ColorPlane":string, "DLP2Config.ColorPaneMapping.Head 4.ColorPane"=→"H4ColorPlane":string, "DLP2Config.ColorPaneMapping.Head 5.ColorPane"=→"H5ColorPlane":string, "DLP2Config.ColorPaneMapping.Head 6.ColorPane"=→"H6ColorPlane":string, "DLP2Config.ColorPaneMapping.Head 1.Material"=w3774:string, "DLP2Config.ColorPaneMapping.Head 2.Material"=w3773:string, "DLP2Config.ColorPaneMapping.Head 3.Material"=w3772:string, "DLP2Config.ColorPaneMapping.Head 4.Material"=w3765:string, "DLP2Config.ColorPaneMapping.Head 5.Material"=w3764:string, "DLP2Config.ColorPaneMapping.Head 6.Material"=w3763:string)  [unwired: 6 out]
        n1351 = property on="Head 1 Material 2" class="Ring (strict)"("RingText.Text"=w3774) -> ()  [unwired: 2 in, 2 out]
        n1352 = property on="Head 2 Material 2" class="Ring (strict)"("RingText.Text"=w3773) -> ()  [unwired: 2 in, 2 out]
        n1353 = property on="Head 3 Material 2" class="Ring (strict)"("RingText.Text"=w3772) -> ()  [unwired: 2 in, 2 out]
        n1354 = property on="Head 4 Material 2" class="Ring (strict)"("RingText.Text"=w3765) -> ()  [unwired: 2 in, 2 out]
        n1355 = property on="Head 5 Material 2" class="Ring (strict)"("RingText.Text"=w3764) -> ()  [unwired: 2 in, 2 out]
        n1356 = property on="Head 6 Material 2" class="Ring (strict)"("RingText.Text"=w3763) -> ()  [unwired: 2 in, 2 out]
        n1357 = call <vilib>:"Add State(s) to Queue__JKI_lib_State_Machine.vi"("State(s) in (\"\")"=w3780) -> ("States Out"=w3779:string)  [unwired: 14 in]
      }
      frame "UI: Read Prime Config" {
        n1358 = Unbundle By Name(w3790) -> ("TopLevel out"=w3781:refnum<class "TopLevel.lvclass">, "Methods:Accessors:ConfigDict"=w3784:T16, "DLP2Config.PrimeModeConfig"=w3786:T27[])
        n1359 = for {
          tunnel: w3786 -> [w3817] mode=indexing
          shift-right: [w3819] -> w3788
          shift-left: w3784 -> [w3814]
          shift-right: [w3818] -> w3787
          shift-left: w3782 -> [w3813]
          (unwired) T27 {"Interval (s)"=0.1, "PurgeDuration (s)"=0.1, "Repeats"=0, "PrimingMode"=enum."Pre-Purge", "Head"=enum."1", "Frequency (Hz)"=0, "PrintWeight"=0.1} ("PrinterMode API Data")
          w3802 = T85 {"Head"=0, "Ink"={"#attributes"={"InkType"="", "ColorPlane"="", "Heat"=0.0, "Meniscus"=0.0, "Recirculation"=FALSE, "PrePrintPurge"=FALSE, "PurgeTime"=0.0, "PurgeCount"=0, "Density"=0.0, "NumberofDrops"=0, "PrintWeight"=0.0, "PrintheadPrime"=FALSE}, "Idle"={"ShortIdle"={"#attributes"={"Heat"=0.0, "Meniscus"=0.0, "Recirculation"=FALSE}}, "LongIdle"={"#attributes"={"Heat"=0.0, "Meniscus"=0.0, "Recirculation"=FALSE}}}}}
          w3810 = T63 {"#attributes"={"HeadNumber"=0, "Material"="", "HeadLocalX"=0.0, "HeadLocalY"=0.0, "HeadRotationAngle"=0.0, "VH2L_Hi"=0.0, "VH2R_Hi"=0.0, "VH1LA_Hi"=0.0, "VH1LB_Hi"=0.0, "VH1RA_Hi"=0.0, "VH1RB_Hi"=0.0, "VH2L_Lo"=0.0, "VH2R_Lo"=0.0, "VH1LA_Lo"=0.0, "VH1LB_Lo"=0.0, "VH1RA_Lo"=0.0, "VH1RB_Lo"=0.0}} ("HeadProperties")
          n1360 = Unbundle By Name(w3817) -> ("Head"=w3795:T18)
          n1361 = Format Into String(w3795) -> (resulting string=w3798:string)  [unwired: 3 in, 1 out]
          n1362 = Concatenate Strings("Head " ("string"), w3798) -> (w3811:string)
          n1363 = call <vilib>:"Get Dynamic CVT Data.vi"("error in (no error)"=w3813, "default value (empty variant)"=w3810, "DataName"=w3811, "dCVT DVR"=w3814) -> ("error out"=w3808:errorcluster, "value"=w3809:variant, "dCVT DVR out"=w3806:T16)  [unwired: 4 in, 1 out]
          n1364 = Variant To Data(error in=w3808, type=w3810, Variant=w3809) -> (data=w3807:T63, error out=w3803:errorcluster)
          n1365 = Unbundle By Name(w3807) -> ("#attributes.Material"=w3804:string)
          n1366 = call <vilib>:"Get Dynamic CVT Data.vi"("error in (no error)"=w3803, "default value (empty variant)"=w3802, "DataName"=w3804, "dCVT DVR"=w3806) -> ("error out"=w3797:errorcluster, "value"=w3801:variant, "dCVT DVR out"=w3805:T16)  [unwired: 4 in, 1 out]
          n1367 = Variant To Data(error in=w3797, type=w3802, Variant=w3801) -> (data=w3800:T85, error out=w3796:errorcluster)
          n1368 = Unbundle By Name(w3800) -> ("Ink.#attributes.PrintWeight"=w3794:dbl)
          n1369 = case shown="\"6\"" w3795 {
            tunnel: w3794 -> [_ w3820 w3821 w3822 w3823 w3824 w3825]
            frame "-1", Default {
            }
            frame "1" {
              n1370 = local write "Weights 1"(w3820) -> ()
            }
            frame "2" {
              n1371 = local write "Weights 2"(w3821) -> ()
            }
            frame "3" {
              n1372 = local write "Weights 3"(w3822) -> ()
            }
            frame "4" {
              n1373 = local write "Weights 4"(w3823) -> ()
            }
            frame "5" {
              n1374 = local write "Weights 5"(w3824) -> ()
            }
            frame "6" {
              n1375 = local write "Weights 6"(w3825) -> ()
            }
          }
          n1376 = Bundle By Name(cluster=w3817, "PrintWeight"=w3794) -> (w3799:T27)
          n1377 = Concatenate Strings("Prime " ("string"), w3798) -> (w3815:string)
          n1378 = call <vilib>:"Set Dynamic CVT Data.vi"("error in (no error)"=w3796, "value"=w3799, "DataName"=w3815, "dCVT DVR"=w3805) -> ("error out"=w3818:errorcluster, "dCVT DVR out"=w3819:T16)  [unwired: 5 in, 1 out]
        }
